vi "calculate_trajectory.vi"(8 "error in (no error)":errorcluster, 11 "TrajectoryAN1106117SinglePoint in":refnum<class "TrajectoryAN1106117SinglePoint.lvclass">) -> (0 "error out":errorcluster, 3 "TrajectoryAN1106117SinglePoint out":refnum<class "TrajectoryAN1106117SinglePoint.lvclass">)   [LabVIEW 2010, in "TrajectoryAN1106117SinglePoint.lvclass"]
uses:
  TrajectoryAN1106117SinglePoint.lvclass
  common/enumerations/x_y_z_enumeration.ctl
  common/enumerations/functional_global_action_enum.ctl
  TrajectoryAN1106117SinglePoint.lvclass/TrajectoryAN1106117SinglePoint.ctl
  common/classes/ImageCollection/ImageCollection/ImageCollection.lvclass
  common/classes/Image/Image/Image.lvclass
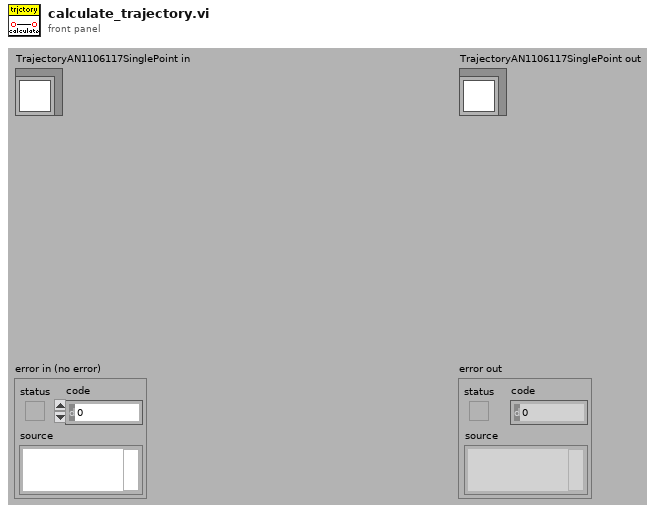
[diagram p1: front panel]
types:
  T1 = typedef "x_y_z_enumeration.ctl" = enum16{"x", "y", "z"}
  T2 = typedef "functional_global_action_enum.ctl" = enum16{"get", "set", "reset"}
  T3 = typedef "ROImicrons_cluster.ctl" = cluster{"Global Rectangle":dbl[unit][], "Contours":cluster{"Contour Type":u32, "ROI Type":u32, "Points":dbl[unit][]}[]}
  T4 = cluster{"Contour Type":u32, "ROI Type":u32, "Points":dbl[unit][]}[]
  T5 = cluster{"Contour Type":u32, "ROI Type":u32, "Points":dbl[unit][]}
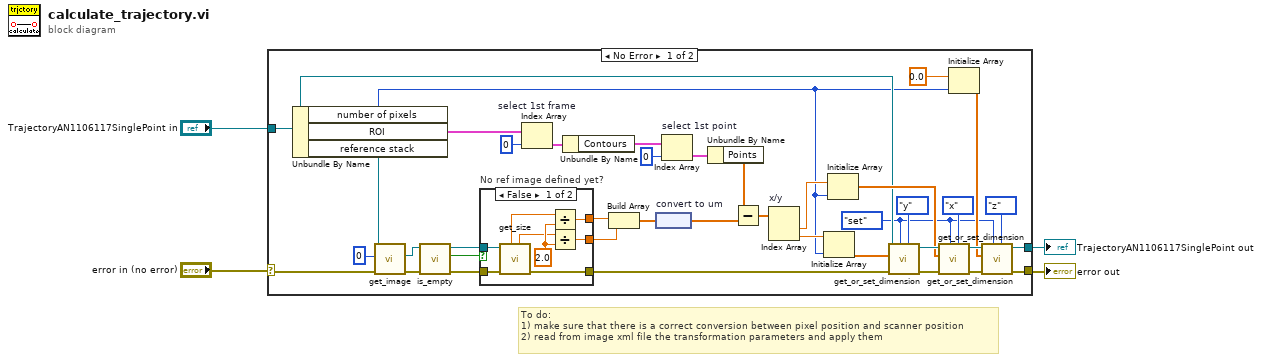
[diagram p0: block diagram]
diagram:
  # "To do:\n1) make sure that there is a correct conversion between pixel position and scanner position\n2) read from image xml file the transformation parameters and apply them"
  n1 = case shown="No Error" "error in (no error)" {
    selector: "error in (no error)" -> [w19 w54]
    tunnel: [w29 w54] -> w3
    tunnel: "TrajectoryAN1106117SinglePoint in" -> [w25 w53]
    tunnel: [w5 w53] -> w4
    frame No Error {
      w6 = functional_global_action_enum."set" ("action")
      n2 = Unbundle By Name(w25) -> ("number of pixels"=w7:i32, "ROI"=w43:T3[], "reference stack"=w20:refnum<class "ImageCollection.lvclass">)
      n3 = call-dynamic "get_image.vi"("error in (no error)"=w19, "index"=0, "ImageCollection in"=w20) -> ("error out"=w22:errorcluster, "Image.lvclass"=w21:refnum<class "Image.lvclass">)  [unwired: 6 in, 1 out]
      n4 = call-dynamic "is_empty.vi"("error in (no error)"=w22, "Image in"=w21) -> ("error out"=w23:errorcluster, "emtpy?"=w17:bool, "Image out"=w18:refnum<class "Image.lvclass">)  [unwired: 7 in]
      n5 = case "No ref image defined yet?" shown="False" w17 {
        tunnel: [w51 w52] -> w8
        tunnel: [w48 _] -> w16
        tunnel: [w46 _] -> w15
        tunnel: w23 -> [w45 w52]
        tunnel: w18 -> [w44 _]
        frame False {
          w50 = 2.0 ("y")
          n6 = call-dynamic "get_size.vi"("error in (no error)"=w45, "Image in"=w44) -> ("error out"=w51:errorcluster, "physical size y"=w47:dbl, "physical size x"=w49:dbl)  [unwired: 2 in, 5 out]
          n7 = Divide(x=w49, y=w50) -> (x/y=w48:dbl)
          n8 = Divide(x=w47, y=w50) -> (x/y=w46:dbl)
        }
        frame True {
        }
      }
      n9 = Index Array "select 1st frame"(array=w43, index=0) -> (element=w41:T3)
      n10 = Unbundle By Name(w41) -> ("Contours"=w39:T4)
      n11 = Build Array(w16, w15) -> (w14:dbl[])
      n12 = node "convert to um"(w14) -> (w13:dbl[unit][])
      n13 = Index Array "select 1st point"(array=w39, index=0) -> (element=w38:T5)
      n14 = Unbundle By Name(w38) -> ("Points"=w12:dbl[unit][])
      n15 = Subtract(x=w12, y=w13) -> (x-y=w11:dbl[unit][])
      n16 = Index Array "x/y"(array=w11) -> (element #1=w10:dbl[unit], element #2=w9:dbl[unit])  [unwired: 2 in]
      n17 = Initialize Array(w9, w7) -> (w33:dbl[unit][])
      n18 = Initialize Array(w10, w7) -> (w32:dbl[unit][])
      n19 = call-dynamic "get_or_set_dimension.vi"("dimension"=x_y_z_enumeration."y", "action"=w6, "error in (no error)"=w8, "pixel values in (single dimension)"=w33, "GenericTrajectory in"=w25) -> ("error out"=w35:errorcluster, "GenericTrajectory out"=w34:refnum<class "TrajectoryAN1106117SinglePoint.lvclass">)  [unwired: 4 in, 1 out]
      n20 = call-dynamic "get_or_set_dimension.vi"("dimension"=x_y_z_enumeration."x", "action"=w6, "error in (no error)"=w35, "pixel values in (single dimension)"=w32, "GenericTrajectory in"=w34) -> ("error out"=w30:errorcluster, "GenericTrajectory out"=w28:refnum<class "TrajectoryAN1106117SinglePoint.lvclass">)  [unwired: 4 in, 1 out]
      n21 = Initialize Array(dbl[unit] 0.0 ("element"), w7) -> (w26:dbl[unit][])
      n22 = call-dynamic "get_or_set_dimension.vi"("dimension"=x_y_z_enumeration."z", "action"=w6, "error in (no error)"=w30, "pixel values in (single dimension)"=w26, "GenericTrajectory in"=w28) -> ("error out"=w29:errorcluster, "GenericTrajectory out"=w5:refnum<class "TrajectoryAN1106117SinglePoint.lvclass">)  [unwired: 4 in, 1 out]
    }
    frame Error {
    }
  }
  "error out" <- w3
  "TrajectoryAN1106117SinglePoint out" <- w4
